vi "Launch Process.vi"(8 "error in (no error)":errorcluster, 11 "DLP2 in":refnum<class "DLP2.lvclass">) -> (0 "error out":errorcluster, 1 "timed out?":bool, 2 "sync from process?":bool, 3 "DLP2 out":refnum<class "DLP2.lvclass">)   [LabVIEW 2022 SP3, in "DLP2.lvclass"]
doc: "Developed by Kevin Thompson\nkevin@thompsonengineering.net\n\nCopyright 2018\nThompson Engineering, LLC"
uses:
  DLP2.lvclass
  Process.vi
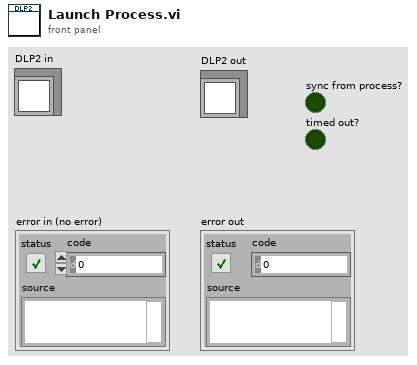
[diagram p1: front panel]
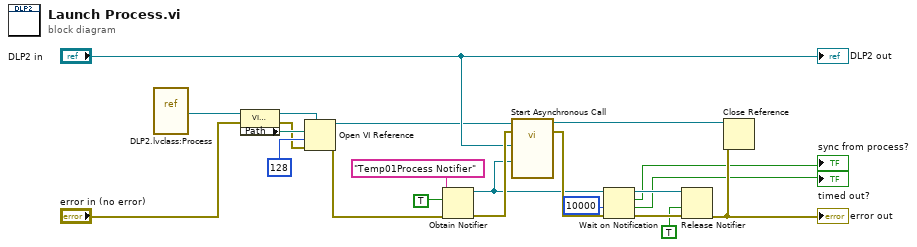
[diagram p0: block diagram]
diagram:
  n1 = vi-ref "DLP2.lvclass:Process.vi"() -> (w9:refnum<vi>)
  n2 = property class="VI (strict)"(reference=w9, error in="error in (no error)") -> (reference out=w7:refnum<vi>, error out=w16:errorcluster, "Path"=w21:path)
  n3 = Open VI Reference(type specifier VI Refnum (for type only)=w7, vi path=w21, options=128, error in (no error)=w16) -> (vi reference=w6:refnum<vi>, error out=w1:errorcluster)  [unwired: 2 in]
  n4 = Obtain Notifier(name (unnamed)="Temp01Process Notifier", notification data type=TRUE, error in (no error)=w1) -> (notifier out=w14:refnum<notifier>, error out=w18:errorcluster)  [unwired: 1 in, 1 out]
  n5 = call-by-ref "Start Asynchronous Call"(reference=w6, error in=w18, "process sync"=w14, "Database in"="DLP2 in") -> (reference out=w11:refnum<vi>, error out=w17:errorcluster)  [unwired: 10 in]
  n6 = Wait on Notification(notifier=w14, timeout in ms (-1)=10000, error in (no error)=w17) -> (notifier out=w12:refnum<notifier>, notification=→"sync from process?":bool, timed out?=→"timed out?":bool, error out=w13:errorcluster)  [unwired: 1 in]
  n7 = Release Notifier(notifier=w12, force destroy? (F)=TRUE, error in (no error)=w13) -> (error out=w22:errorcluster)  [unwired: 2 out]
  "error out" <- w22
  n8 = Close Reference(reference=w11, error in (no error)=w22) -> ()  [unwired: 1 out]
  "DLP2 out" <- "DLP2 in"
